vi "Read.vi"(8 "error in (no error)":errorcluster, 11 "TDMS Group in":refnum<class "Group.lvclass">) -> (0 "error out":errorcluster, 1 "Group Properties":refnum<class "Variant.lvclass">, 2 "Channels":refnum<class "Channel.lvclass">[](array[class]), 3 "Group Name":string)   [LabVIEW 2020, in "TDMS.lvlib" / "Group.lvclass"]
doc: "Read Group Name, Channels and Properties."
uses:
  Group.lvclass
  TDMS Channel/Channel.lvclass
  PPL/HDH.Data.Generic.lvlibp/Generic Data/Variant/Variant.lvclass
  Group.lvclass/Group.ctl
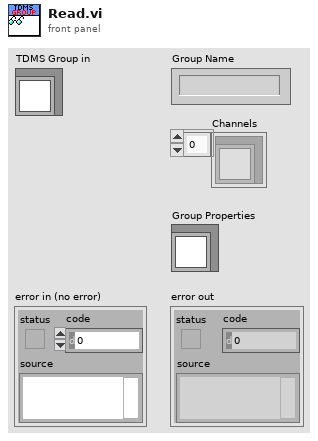
[diagram p1: front panel]
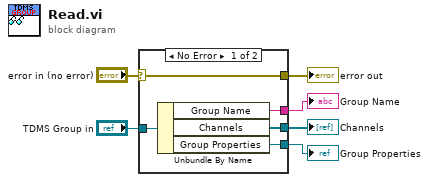
[diagram p0: block diagram]
diagram:
  n1 = case shown="No Error" "error in (no error)" {
    selector: "error in (no error)" -> [w11 w12]
    tunnel: [w11 w12] -> w5
    tunnel: "TDMS Group in" -> [w10 _]
    tunnel: [w9 _] -> w3
    tunnel: [w8 _] -> w2
    tunnel: [w7 _] -> w1
    frame No Error {
      n2 = Unbundle By Name(w10) -> ("Group Name"=w9:string, "Channels"=w8:refnum<class "Channel.lvclass">[], "Group Properties"=w7:refnum<class "Variant.lvclass">)
    }
    frame Error {
    }
  }
  "error out" <- w5
  "Group Name" <- w3
  "Channels" <- w2
  "Group Properties" <- w1
